vi "filtered.data.event.get.vi"(11 "manager_daemon in":refnum<class "manager_daemon.lvclass">) -> (2 "filter data event":refnum<user-event>, 3 "manager_daemon out":refnum<class "manager_daemon.lvclass">)   [LabVIEW 2024, in "manager_daemon.lvclass"]
uses:
  manager_daemon.lvclass
  CV_Shared_Library/volume.object--cluster.ctl
  CV_Shared_Library/volume.type--enum.ctl
  TypeDefs/issue.display--cluster.ctl
  manager_daemon.lvclass/manager_daemon.ctl
  CV_Shared_Library/CV_Shared_Library.lvlib
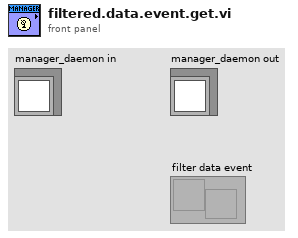
[diagram p1: front panel]
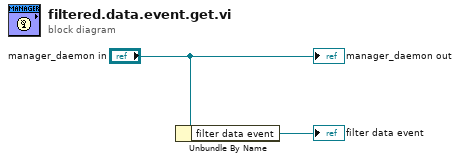
[diagram p0: block diagram]
diagram:
  n1 = Unbundle By Name("manager_daemon in") -> ("filter data event"=→"filter data event":refnum<user-event>)
  "manager_daemon out" <- "manager_daemon in"
